vi "Configure Scale.vi"(0 "VISA resource name":refnum<visa-resource-name>, 1 "Channel (1)":i32=1, 2 "Trace (1)":i32=1, 5 "Number of Division (10)":i32=10, 7 "Scale Per Division (10.0)":dbl=10.0 format="%^.2e", 9 "Value Graticule Line (0.0)":dbl format="%^.2e", 11 "error in (no error)":errorcluster, 12 "Reference Graticule Line (5)":i32=5) -> (4 "VISA resource name out":refnum<visa-resource-name>, 15 "error out":errorcluster)   [LabVIEW 2012, in "Tektronix TTR500 Series.lvlib"]
doc: "This VI configures display scale."
uses:
  <instrlib>/Tektronix TTR500 Series/Tektronix TTR500 Series.lvlib
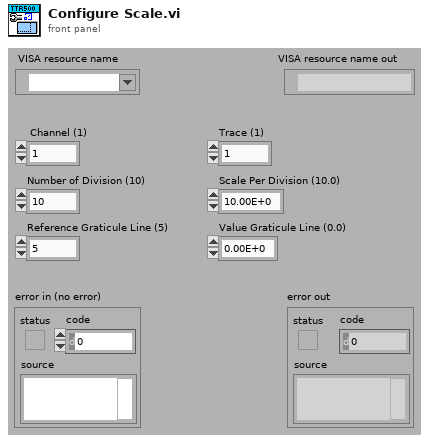
[diagram p1: front panel]
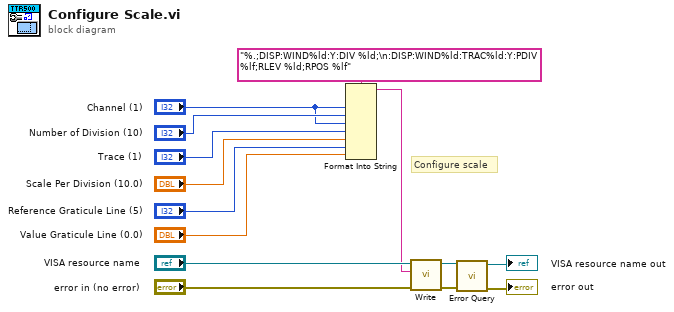
[diagram p0: block diagram]
diagram:
  # "Configure scale"
  n1 = Format Into String(format string="%.;DISP:WIND%ld:Y:DIV %ld;\n:DISP:WIND%ld:TRAC%ld:Y:PDIV %lf;RLEV %ld;RPOS %lf", "Channel (1)", "Number of Division (10)", "Channel (1)", "Trace (1)", "Scale Per Division (10.0)", "Reference Graticule Line (5)", "Value Graticule Line (0.0)") -> (resulting string=w11:string)  [unwired: 2 in, 1 out]
  n2 = call <instrlib>:"Write.vi"("error in (no error)"="error in (no error)", "String ()"=w11, "VISA resource name"="VISA resource name") -> ("error out"=w3:errorcluster, "VISA resource name out"=w4:refnum<visa-resource-name>)  [unwired: 6 in, 1 out]
  n3 = call <instrlib>:"Error Query.vi"("error in (no error)"=w3, "VISA resource name"=w4) -> ("error out"=→"error out":errorcluster, "VISA resource name out"=→"VISA resource name out":refnum<visa-resource-name>)  [unwired: 6 in, 2 out]
